vi "Begin.vi"(11 "Image Size":T1=enum."160x120") -> (0 "error out":errorcluster)   [LabVIEW 2011]
doc: "Called before other user functions, this VI is expected to open initial I/O refnums, load in file data, and do all program initialization. Notice that the <B>error out</B> terminal is simply used for data flow. Wiring it to other structures or subVIs ensures that this VI runs first."
uses:
  <vilib>/Rock Robotics/WPI/Camera/WPI_CameraImageSize.ctl
  <vilib>/Rock Robotics/SystemInterfaces/DIO/FPGA_DIOPWMChannel.ctl
  <vilib>/Rock Robotics/WPI/Joystick/WPI_JoystickDeviceEnum.ctl
  <vilib>/Rock Robotics/WPI/Camera/WPI_CameraWhite Balance Values.ctl
  <vilib>/Rock Robotics/WPI/Camera/WPI_CameraExposure Values.ctl
  <vilib>/Rock Robotics/WPI/Camera/WPI_CameraFrameRate.ctl
  <vilib>/Rock Robotics/SystemInterfaces/Typedef/FPGA_TypedefDigitalModule.ctl
  <vilib>/Rock Robotics/SystemInterfaces/Typedef/FPGA_TypedefAnalogModule.ctl
  <vilib>/Rock Robotics/SystemInterfaces/AI/FPGA_AIChannel.ctl
  <vilib>/Rock Robotics/SystemInterfaces/DIO/FPGA_DIOChannel.ctl
  <vilib>/Rock Robotics/SystemInterfaces/Typedef/FPGA_TypedefAnalogModuleForGyro.ctl
  <vilib>/Rock Robotics/SystemInterfaces/AI/FPGA_AIGyroChannel.ctl
  Common/ADXL345 I2C Range.ctl
  <vilib>/Rock Robotics/SystemInterfaces/DIO/FPGA_DIORelayChannel.ctl
  <vilib>/Rock Robotics/WPI/RobotDrive/WPI_RobotDriveOpen4MotorWithJaguar.vi
  <vilib>/Rock Robotics/WPI/MotorControl/WPI_MotorControlOpen Jaguar.vi
  <vilib>/Rock Robotics/WPI/Counter/WPI_CounterDigitalInputToDigitalSource.vi
  <vilib>/Rock Robotics/WPI/Counter/WPI_CounterOpen UpDown Mode.vi
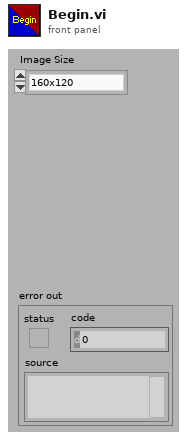
[diagram p1: front panel]
types:
  T1 = typedef "WPI_CameraImageSize.ctl" = enum16{"640x480", "320x240", "160x120"}
  T2 = typedef "FPGA_DIORelayChannel.ctl" = enum8{"Relay 1", "Relay 2", "Relay 3", "Relay 4", "Relay 5", "Relay 6", "Relay 7", "Relay 8", "Invalid"}
  T3 = typedef "FPGA_TypedefDigitalModule.ctl" = enum16{"Digital Module 1", "Digital Module 2"}
  T4 = typedef "FPGA_DIOChannel.ctl" = enum8{"DIO 1", "DIO 2", "DIO 3", "DIO 4", "DIO 5", "DIO 6", "DIO 7", "DIO 8", "DIO 9", "DIO 10", "DIO 11", "DIO 12", "DIO 13", "DIO 14", "Invalid"}
  T5 = typedef "FPGA_AIChannel.ctl" = enum8{"AI 1", "AI 2", "AI 3", "AI 4", "AI 5", "AI 6", "AI 7", "AI 8", "Invalid"}
  T6 = typedef "FPGA_TypedefAnalogModule.ctl" = enum16{"Analog Module 1", "Analog Module 2"}
  T7 = typedef "FPGA_DIOPWMChannel.ctl" = enum8{"PWM 1", "PWM 2", "PWM 3", "PWM 4", "PWM 5", "PWM 6", "PWM 7", "PWM 8", "PWM 9", "PWM 10", "Invalid"}
  T8 = typedef "ADXL345 I2C Range.ctl" = u8
  T9 = typedef "FPGA_AIGyroChannel.ctl" = enum8{"AI 1", "AI 2", "Invalid"}
  T10 = typedef "FPGA_TypedefAnalogModuleForGyro.ctl" = enum16{"Analog Module 1"}
  T11 = typedef "WPI_JoystickDeviceEnum.ctl" = enum16{"USB 1", "USB 2", "USB 3", "USB 4", "Kinect 1", "Kinect 2"}
  T12 = typedef "WPI_CameraFrameRate.ctl" = u32
  T13 = typedef "WPI_CameraExposure Values.ctl" = enum16{"Auto", "Flicker-free 50 Hz", "Flicker-free 60 Hz", "Hold current"}
  T14 = typedef "WPI_CameraWhite Balance Values.ctl" = enum16{"Auto", "Fixed indoor", "Fixed outdoor 1", "Fixed outdoor 2", "Fixed fluorescent 1", "Fixed fluorescent 2", "Hold current"}
  T15 = typedef "WPI_DigitalInputDevRef.ctl" = cluster{"DevStatus":errorcluster, "DIO Channel":T4, "Digital Module":T3}
  T16 = typedef "WPI_JoystickDevRef.ctl" = cluster{"Device":T11}
  T17 = typedef "WPI_AnalogChannelDevRef.ctl" = cluster{"DevStatus":errorcluster, "Analog Module":T6, "Analog Channel":T5}
  T18 = typedef "WPI_RobotDriveDevRef.ctl" = cluster{"DevStatus":errorcluster, "Motors[]":T19[], "Square Inputs":bool, "Max Output":dbl, "Isochronous":bool}
  T19 = typedef "WPI_MotorControlDeviceRef.ctl" = cluster{"DeviceStatus":errorcluster, "Type":enum16{"PWM", "CAN"}, "PWM":cluster{"Digital Module":T3, "PWM Channel":T7, "DeadBand":T20}, "CAN":cluster{"Device Number":u8, "Control Mode":T21, "Semaphore":T22, "Max Vout":dbl}, "Invert":bool, "TransformRef":T23, "InvTransformRef":T23}
  T20 = typedef "WPI_PWMDeadband.ctl" = cluster{"Name":string, "maxPositivePwm":i32, "minPositivePwm":i32, "centerPwm":i32, "maxNegativePwm":i32, "minNegativePwm":i32, "angularRange":u16}
  T21 = typedef "WPI_CANJaguar_ControlMode.ctl" = enum8{"Percent VBus", "Current", "Speed", "Position", "Voltage"}
  T22 = typedef "Semaphore RefNum" = refnum<k1>
  T23 = typedef "WPI_PWMTransform_ConPane.ctl" = refnum<vi>
  T24 = typedef "WPI_GyroDevRef.ctl" = cluster{"DevStatus":errorcluster, "Analog Module":T6, "Analog Channel":T5, "Offset":dbl, "Gain (VoltsPerDegree/Second)":dbl}
  T25 = typedef "WPI_I2CDevRef.ctl" = cluster{"DevStatus":errorcluster, "Digital Module":T3, "Device Address":u8}
  T26 = typedef "WPI_RelayDevRef.ctl" = cluster{"DevStatus":errorcluster, "Relay Channel":T2, "Digital Module":T3, "Relay Direction":T27}
  T27 = typedef "WPI_RelayDirection.ctl" = enum16{"Both directions", "Forward only", "Reverse only"}
  T28 = typedef "FPGA_CounterEncoderSourceConvertionLVSourceType.ctl" = cluster{"DevStatus":errorcluster, "AnalogTriggerMode?":bool, "DigitalMode":cluster{"Digital Module":T3, "DIO Channel":T29}, "AnalogTriggerMode":cluster{"AnalogTriggerIndex":T30, "OutputType":T31}}
  T29 = typedef "FPGA_DIODigitalSourceChannel.ctl" = enum8{"DIO 1", "DIO 2", "DIO 3", "DIO 4", "DIO 5", "DIO 6", "DIO 7", "DIO 8", "DIO 9", "DIO 10", "DIO 11", "DIO 12", "DIO 13", "DIO 14", "Disabled"}
  T30 = typedef "FPGA_AnalogTriggerIndex.ctl" = enum8{"Trig 0", "Trig 1", "Trig 2", "Trig 3", "Trig 4", "Trig 5", "Trig 6", "Trig 7", "Invalid"}
  T31 = typedef "FPGA_AnalogTriggerOutType.ctl" = enum16{"InWindow", "TriggerState", "Rising", "Falling"}
  T32 = typedef "WPI_EncoderDevRef.ctl" = cluster{"DevStatus":errorcluster, "EncoderIndex":T33, "CounterIndex":T34, "DistancePerCount":dbl, "Decoding Type":T35}
  T33 = typedef "FPGA_EncoderIdx.ctl" = enum8{"Enc 0", "Enc 1", "Enc 2", "Enc 3", "Invalid"}
  T34 = typedef "FPGA_CounterCtrSystemIndex.ctl" = enum8{"Ctr 0", "Ctr 1", "Ctr 2", "Ctr 3", "Ctr 4", "Ctr 5", "Ctr 6", "Ctr 7", "Invalid"}
  T35 = typedef "WPI_EncoderType.ctl" = enum16{"1x", "2x", "4x"}
  T36 = typedef "WPI_CounterDevRef.ctl" = cluster{"DevStatus":errorcluster, "CntIndex":T34}
  T37 = typedef "WPI_CameraDevRef.ctl" = cluster{"Camera Address":string, "CameraStatus":errorcluster, "Acquire Image Notifier":refnum<notifier>}
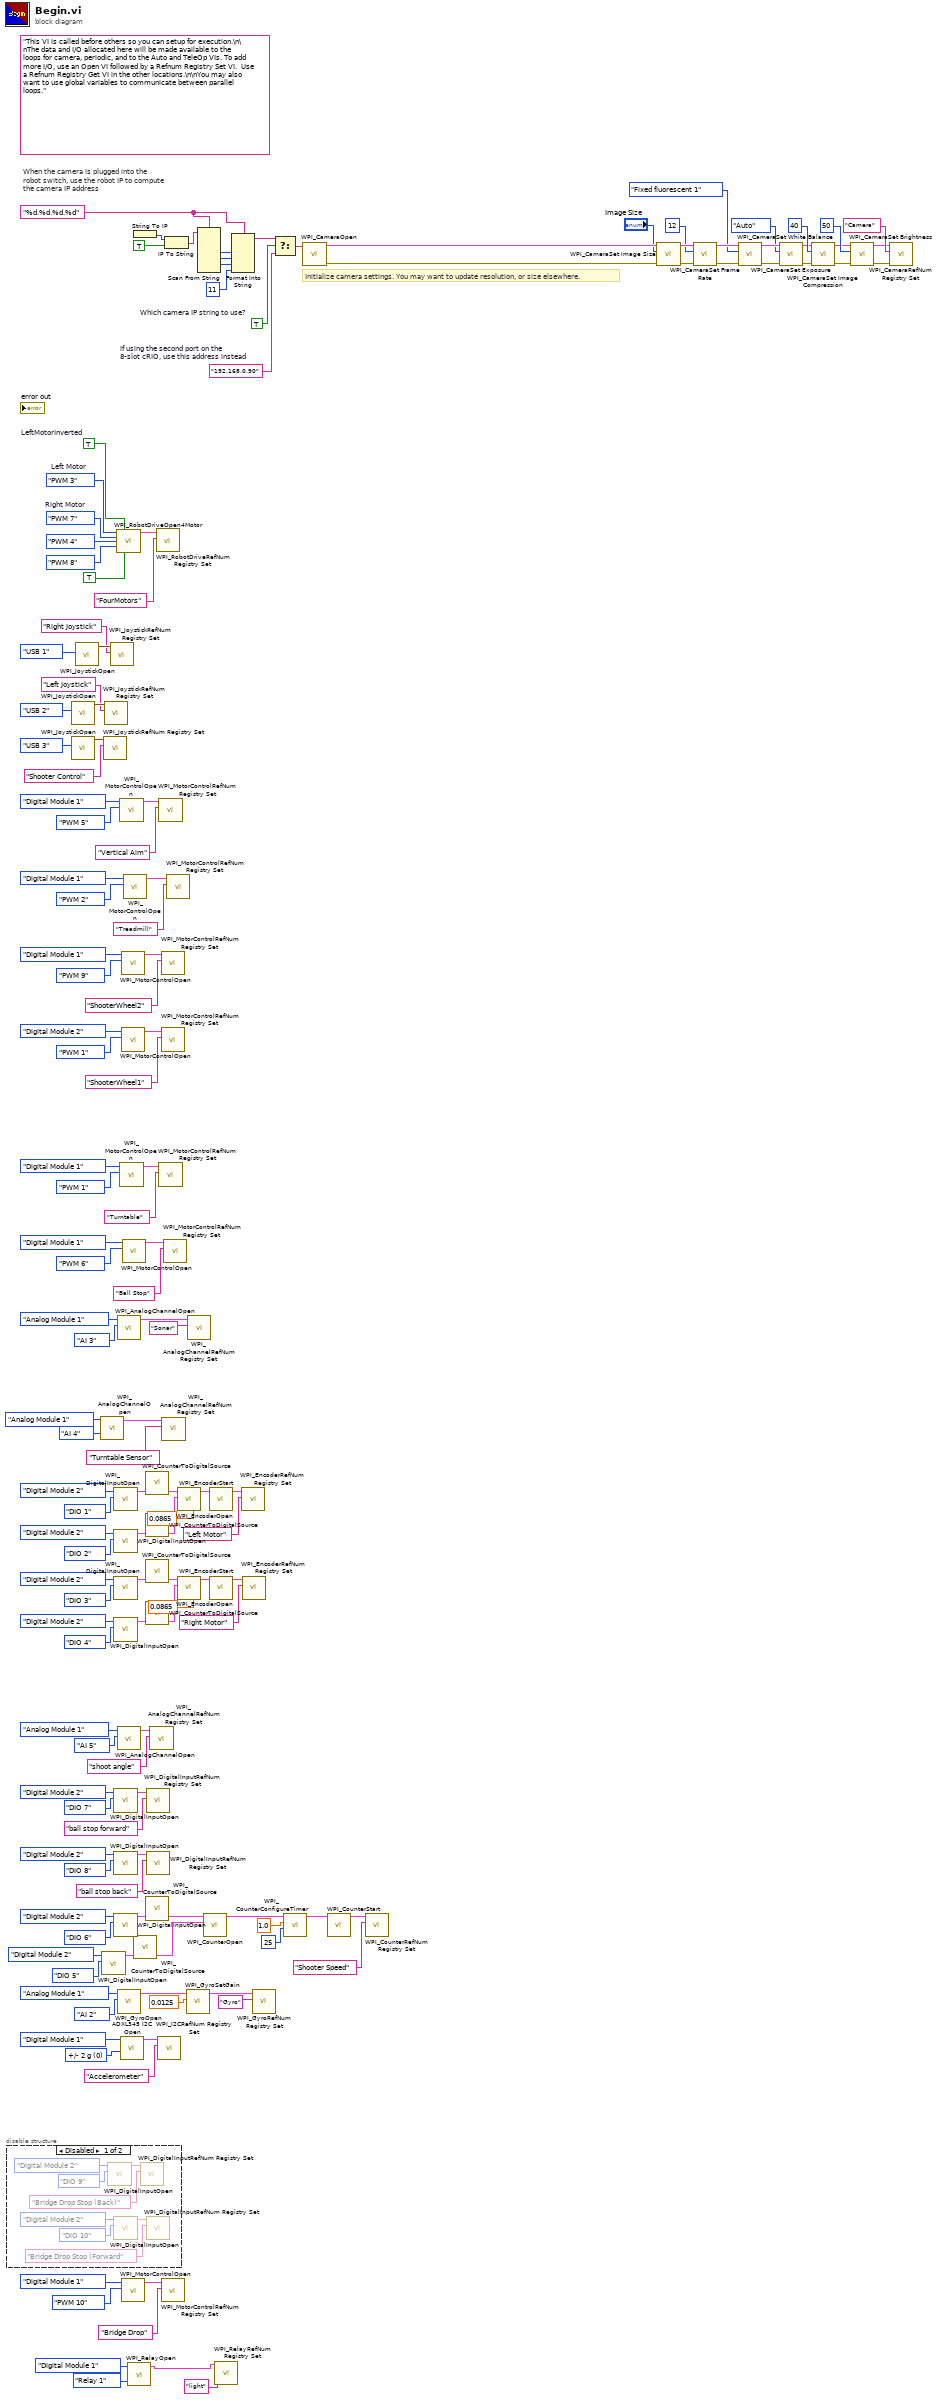
[diagram p0: block diagram]
diagram:
  w23 = T8 0 items=["+/- 2 g", "+/- 4 g", "+/- 8 g", "+/- 16 g"] ("Range")
  w110 = TRUE  # Which camera IP string to use?
  w114 = "%d.%d.%d.%d" ("format string")
  (unwired) "This VI is called before others so you can setup for execution.\n\nThe data and I/O allocated here will be made available to the loops for camera, periodic, and to the Auto and TeleOp VIs. To add more I/O, use an Open VI followed by a Refnum Registry Set VI.  Use a Refnum Registry Get VI in the other locations.\n\nYou may also want to use global variables to communicate between parallel loops."
  w126 = FPGA_DIOPWMChannel."PWM 7"  # Right Motor
  w127 = FPGA_DIOPWMChannel."PWM 3"  # Left Motor
  w111 = "192.168.0.90"  # If using the second port on the 8-slot cRIO, use this address instead
  w150 = TRUE  # LeftMotorInverted
  # "When the camera is plugged into the\nrobot switch, use the robot IP to compute\nthe camera IP address"
  # "Initialize camera settings. You may want to update resolution, or size elsewhere."
  n1 = disable-structure shown="Disabled" {
    frame Disabled {
      n2 = call <vilib>:"WPI_DigitalInputOpen.vi"("DIO Channel"=FPGA_DIOChannel."DIO 9", "Digital Module (Module 1)"=FPGA_TypedefDigitalModule."Digital Module 2") -> ("DigitalInputDevRef"=w151:T15)  [unwired: 8 in, 1 out]
      n3 = call <vilib>:"WPI_DigitalInputOpen.vi"("DIO Channel"=FPGA_DIOChannel."DIO 10", "Digital Module (Module 1)"=FPGA_TypedefDigitalModule."Digital Module 2") -> ("DigitalInputDevRef"=w158:T15)  [unwired: 8 in, 1 out]
      n4 = call <vilib>:"WPI_DigitalInputRefNum Registry Set.vi"("refnum name"="Bridge Drop Stop (Back)", "DigitalInputDevRef"=w151) -> ()  [unwired: 8 in, 2 out]
      n5 = call <vilib>:"WPI_DigitalInputRefNum Registry Set.vi"("refnum name"="Bridge Drop Stop (Forward", "DigitalInputDevRef"=w158) -> ()  [unwired: 8 in, 2 out]
    }
    frame Enabled {
    }
  }
  n6 = call <vilib>:"WPI_JoystickOpen.vi"("JoystickDevice"=WPI_JoystickDeviceEnum."USB 2") -> ("JoystickDevRef"=w109:T16)  [unwired: 10 in]
  n7 = call <vilib>:"WPI_JoystickOpen.vi"("JoystickDevice"=WPI_JoystickDeviceEnum."USB 3") -> ("JoystickDevRef"=w105:T16)  [unwired: 10 in]
  n8 = call <vilib>:"WPI_JoystickOpen.vi"("JoystickDevice"=WPI_JoystickDeviceEnum."USB 1") -> ("JoystickDevRef"=w146:T16)  [unwired: 10 out]
  n9 = call <vilib>:"WPI_AnalogChannelOpen.vi"("Analog Channel"=FPGA_AIChannel."AI 4", "Analog Module (Module 1)"=FPGA_TypedefAnalogModule."Analog Module 1") -> ("AIDeviceRef"=w14:T17)  [unwired: 8 in, 1 out]
  n10 = call <vilib>:"WPI_DigitalInputOpen.vi"("DIO Channel"=FPGA_DIOChannel."DIO 5", "Digital Module (Module 1)"=FPGA_TypedefDigitalModule."Digital Module 2") -> ("DigitalInputDevRef"=w10:T15)  [unwired: 8 in, 1 out]
  n11 = call <vilib>:"WPI_JoystickRefNum Registry Set.vi"("refnum name"="Shooter Control", "JoystickDevRef"=w105) -> ()  [unwired: 8 in, 2 out]
  n12 = call <vilib>:"WPI_JoystickRefNum Registry Set.vi"("refnum name"="Left Joystick", "JoystickDevRef"=w109) -> ()  [unwired: 8 in, 2 out]
  n13 = call <vilib>:"WPI_JoystickRefNum Registry Set.vi"("refnum name"="Right Joystick", "JoystickDevRef"=w146) -> ()  [unwired: 1 in, 9 out]
  n14 = call <vilib>:"WPI_DigitalInputOpen.vi"("DIO Channel"=FPGA_DIOChannel."DIO 1", "Digital Module (Module 1)"=FPGA_TypedefDigitalModule."Digital Module 2") -> ("DigitalInputDevRef"=w67:T15)  [unwired: 8 in, 1 out]
  n15 = call <vilib>:"WPI_DigitalInputOpen.vi"("DIO Channel"=FPGA_DIOChannel."DIO 2", "Digital Module (Module 1)"=FPGA_TypedefDigitalModule."Digital Module 2") -> ("DigitalInputDevRef"=w68:T15)  [unwired: 8 in, 1 out]
  n16 = call <vilib>:"WPI_DigitalInputOpen.vi"("DIO Channel"=FPGA_DIOChannel."DIO 3", "Digital Module (Module 1)"=FPGA_TypedefDigitalModule."Digital Module 2") -> ("DigitalInputDevRef"=w69:T15)  [unwired: 8 in, 1 out]
  n17 = call <vilib>:"WPI_DigitalInputOpen.vi"("DIO Channel"=FPGA_DIOChannel."DIO 4", "Digital Module (Module 1)"=FPGA_TypedefDigitalModule."Digital Module 2") -> ("DigitalInputDevRef"=w70:T15)  [unwired: 8 in, 1 out]
  n18 = call <vilib>:"WPI_DigitalInputOpen.vi"("DIO Channel"=FPGA_DIOChannel."DIO 7", "Digital Module (Module 1)"=FPGA_TypedefDigitalModule."Digital Module 2") -> ("DigitalInputDevRef"=w49:T15)  [unwired: 8 in, 1 out]
  n19 = call <vilib>:"WPI_DigitalInputOpen.vi"("DIO Channel"=FPGA_DIOChannel."DIO 8", "Digital Module (Module 1)"=FPGA_TypedefDigitalModule."Digital Module 2") -> ("DigitalInputDevRef"=w50:T15)  [unwired: 8 in, 1 out]
  n20 = call <vilib>:"WPI_DigitalInputOpen.vi"("DIO Channel"=FPGA_DIOChannel."DIO 6", "Digital Module (Module 1)"=FPGA_TypedefDigitalModule."Digital Module 2") -> ("DigitalInputDevRef"=w42:T15)  [unwired: 8 in, 1 out]
  n21 = call-poly <vilib>:"WPI_RobotDriveOpen4Motor.vi"("Rear Left Motor"=w127, "Rear Left Motor Inverted"=w150, "Rear Right Motor"=w126, "Front Left Motor"=FPGA_DIOPWMChannel."PWM 4", "Front Right Motor"=FPGA_DIOPWMChannel."PWM 8", "Front Left Motor Inverted"=TRUE) -> ("RobotDriveDevRef"=w148:T18)  [unwired: 8 in, 1 out]
  n22 = call <vilib>:"WPI_AnalogChannelOpen.vi"("Analog Channel"=FPGA_AIChannel."AI 3", "Analog Module (Module 1)"=FPGA_TypedefAnalogModule."Analog Module 1") -> ("AIDeviceRef"=w80:T17)  [unwired: 8 in, 1 out]
  n23 = call <vilib>:"WPI_AnalogChannelOpen.vi"("Analog Channel"=FPGA_AIChannel."AI 5", "Analog Module (Module 1)"=FPGA_TypedefAnalogModule."Analog Module 1") -> ("AIDeviceRef"=w52:T17)  [unwired: 8 in, 1 out]
  n24 = call <vilib>:"WPI_GyroOpen.vi"("Analog Channel"=FPGA_AIGyroChannel."AI 2", "Analog Module (Module 1)"=FPGA_TypedefAnalogModuleForGyro."Analog Module 1") -> ("GyroDevRef"=w32:T24)  [unwired: 4 in, 5 out]
  n25 = call-poly <vilib>:"WPI_MotorControlOpen.vi"("PWM Channel"=FPGA_DIOPWMChannel."PWM 5", "Digital Module (Module 1)"=FPGA_TypedefDigitalModule."Digital Module 1") -> ("MotorControlDeviceRef"=w100:T19)  [unwired: 8 in, 1 out]
  n26 = call-poly <vilib>:"WPI_MotorControlOpen.vi"("PWM Channel"=FPGA_DIOPWMChannel."PWM 1", "Digital Module (Module 1)"=FPGA_TypedefDigitalModule."Digital Module 1") -> ("MotorControlDeviceRef"=w82:T19)  [unwired: 8 in, 1 out]
  n27 = call "ADXL345 I2C Open.vi"("Range"=w23, "DIO Module (Slot 4)"=FPGA_TypedefDigitalModule."Digital Module 1") -> ("I2CDevRef"=w26:T25)  [unwired: 2 in, 7 out]
  n28 = call-poly <vilib>:"WPI_MotorControlOpen.vi"("PWM Channel"=FPGA_DIOPWMChannel."PWM 9", "Digital Module (Module 1)"=FPGA_TypedefDigitalModule."Digital Module 1") -> ("MotorControlDeviceRef"=w92:T19)  [unwired: 8 in, 1 out]
  n29 = call-poly <vilib>:"WPI_MotorControlOpen.vi"("PWM Channel"=FPGA_DIOPWMChannel."PWM 1", "Digital Module (Module 1)"=FPGA_TypedefDigitalModule."Digital Module 2") -> ("MotorControlDeviceRef"=w91:T19)  [unwired: 8 in, 1 out]
  n30 = call-poly <vilib>:"WPI_MotorControlOpen.vi"("PWM Channel"=FPGA_DIOPWMChannel."PWM 10", "Digital Module (Module 1)"=FPGA_TypedefDigitalModule."Digital Module 1") -> ("MotorControlDeviceRef"=w18:T19)  [unwired: 8 in, 1 out]
  n31 = call-poly <vilib>:"WPI_MotorControlOpen.vi"("PWM Channel"=FPGA_DIOPWMChannel."PWM 6", "Digital Module (Module 1)"=FPGA_TypedefDigitalModule."Digital Module 1") -> ("MotorControlDeviceRef"=w22:T19)  [unwired: 8 in, 1 out]
  n32 = call-poly <vilib>:"WPI_MotorControlOpen.vi"("PWM Channel"=FPGA_DIOPWMChannel."PWM 2", "Digital Module (Module 1)"=FPGA_TypedefDigitalModule."Digital Module 1") -> ("MotorControlDeviceRef"=w96:T19)  [unwired: 8 in, 1 out]
  n33 = call <vilib>:"WPI_RelayOpen.vi"("Relay Channel"=FPGA_DIORelayChannel."Relay 1", "Digital Module (Module 1)"=FPGA_TypedefDigitalModule."Digital Module 1") -> ("RelayDevRef"=w6:T26)  [unwired: 8 in, 1 out]
  n34 = String To IP() -> (0:w121:u32)  [unwired: 1 in]
  n35 = call-poly <vilib>:"WPI_CounterToDigitalSource.vi"("DigitalInputDevRef"=w10) -> ("Digital Source"=w7:T28)  [unwired: 6 in]
  n36 = call-poly <vilib>:"WPI_CounterToDigitalSource.vi"("DigitalInputDevRef"=w67) -> ("Digital Source"=w76:T28)  [unwired: 6 in]
  n37 = call-poly <vilib>:"WPI_CounterToDigitalSource.vi"("DigitalInputDevRef"=w68) -> ("Digital Source"=w75:T28)  [unwired: 6 in]
  n38 = call-poly <vilib>:"WPI_CounterToDigitalSource.vi"("DigitalInputDevRef"=w69) -> ("Digital Source"=w72:T28)  [unwired: 6 in]
  n39 = call-poly <vilib>:"WPI_CounterToDigitalSource.vi"("DigitalInputDevRef"=w70) -> ("Digital Source"=w71:T28)  [unwired: 6 in]
  n40 = call-poly <vilib>:"WPI_CounterToDigitalSource.vi"("DigitalInputDevRef"=w42) -> ("Digital Source"=w39:T28)  [unwired: 6 in]
  n41 = call <vilib>:"WPI_DigitalInputRefNum Registry Set.vi"("refnum name"="ball stop forward", "DigitalInputDevRef"=w49) -> ()  [unwired: 8 in, 2 out]
  n42 = call <vilib>:"WPI_DigitalInputRefNum Registry Set.vi"("refnum name"="ball stop back", "DigitalInputDevRef"=w50) -> ()  [unwired: 8 in, 2 out]
  n43 = call <vilib>:"WPI_AnalogChannelRefNum Registry Set.vi"("refnum name"="shoot angle", "AIDeviceRef"=w52) -> ()  [unwired: 8 in, 2 out]
  n44 = call <vilib>:"WPI_RobotDriveRefNum Registry Set.vi"("refnum name"="FourMotors", "RobotDriveDevRef"=w148) -> ()  [unwired: 1 in, 9 out]
  n45 = call <vilib>:"WPI_I2CRefNum Registry Set.vi"("refnum name"="Accelerometer", "I2CDevRef"=w26) -> ()  [unwired: 8 in, 2 out]
  n46 = call <vilib>:"WPI_MotorControlRefNum Registry Set.vi"("refnum name"="Vertical Aim", "MotorControlDevRef"=w100) -> ()  [unwired: 8 in, 2 out]
  n47 = call <vilib>:"WPI_MotorControlRefNum Registry Set.vi"("refnum name"="Turntable", "MotorControlDevRef"=w82) -> ()  [unwired: 8 in, 2 out]
  n48 = call <vilib>:"WPI_MotorControlRefNum Registry Set.vi"("refnum name"="ShooterWheel2", "MotorControlDevRef"=w92) -> ()  [unwired: 8 in, 2 out]
  n49 = call <vilib>:"WPI_MotorControlRefNum Registry Set.vi"("refnum name"="ShooterWheel1", "MotorControlDevRef"=w91) -> ()  [unwired: 8 in, 2 out]
  n50 = call <vilib>:"WPI_MotorControlRefNum Registry Set.vi"("refnum name"="Bridge Drop", "MotorControlDevRef"=w18) -> ()  [unwired: 8 in, 2 out]
  n51 = call <vilib>:"WPI_AnalogChannelRefNum Registry Set.vi"("refnum name"="Turntable Sensor", "AIDeviceRef"=w14) -> ()  [unwired: 8 in, 2 out]
  n52 = call <vilib>:"WPI_MotorControlRefNum Registry Set.vi"("refnum name"="Ball Stop", "MotorControlDevRef"=w22) -> ()  [unwired: 8 in, 2 out]
  n53 = IP To String(1:TRUE ("dot notation? (F)"), 2:w121) -> (0:w119:string)
  n54 = call <vilib>:"WPI_MotorControlRefNum Registry Set.vi"("refnum name"="Treadmill", "MotorControlDevRef"=w96) -> ()  [unwired: 8 in, 2 out]
  n55 = call <vilib>:"WPI_EncoderOpen.vi"("DistancePerCount"=0.0865, "BSource"=w75, "ASource"=w76) -> ("EncoderDevRef"=w73:T32)  [unwired: 7 in, 1 out]
  n56 = call <vilib>:"WPI_EncoderOpen.vi"("DistancePerCount"=0.0865, "BSource"=w71, "ASource"=w72) -> ("EncoderDevRef"=w74:T32)  [unwired: 7 in, 1 out]
  n57 = call <vilib>:"WPI_GyroSetGain.vi"("Gain (VoltsPerDegree/Second)"=0.0125, "GyroDevRef"=w32) -> ("GyroDevRef"=w28:T24)  [unwired: 1 in, 8 out]
  n58 = call <vilib>:"WPI_AnalogChannelRefNum Registry Set.vi"("refnum name"="Sonar", "AIDeviceRef"=w80) -> ()  [unwired: 8 in, 2 out]
  n59 = Scan From String(format string=w114, input string=w119) -> (output 1=w118:i32, output 2=w117:i32, output 3=w116:i32)  [unwired: 7 in, 3 out]
  n60 = call-poly <vilib>:"WPI_CounterOpen.vi"("Down Source"=w7, "Up Source"=w39) -> ("CounterDevRef"=w33:T36)  [unwired: 8 in, 1 out]
  n61 = call <vilib>:"WPI_EncoderStart.vi"("EncoderDevRef"=w73) -> ("EncoderDevRef"=w57:T32)  [unwired: 9 in, 1 out]
  n62 = call <vilib>:"WPI_EncoderStart.vi"("EncoderDevRef"=w74) -> ("EncoderDevRef"=w58:T32)  [unwired: 9 in, 1 out]
  n63 = call <vilib>:"WPI_RelayRefNum Registry Set.vi"("refnum name"="light", "RelayDevRef"=w6) -> ()  [unwired: 8 in, 2 out]
  n64 = Format Into String(format string=w114, w118, w117, w116, 11 ("Compression")) -> (resulting string=w112:string)  [unwired: 2 in, 1 out]
  n65 = call <vilib>:"WPI_EncoderRefNum Registry Set.vi"("refnum name"="Left Motor", "EncoderDevRef"=w57) -> ()  [unwired: 8 in, 2 out]
  n66 = call <vilib>:"WPI_EncoderRefNum Registry Set.vi"("refnum name"="Right Motor", "EncoderDevRef"=w58) -> ()  [unwired: 8 in, 2 out]
  n67 = call <vilib>:"WPI_GyroRefNum Registry Set.vi"("refnum name"="Gyro", "GyroDevRef"=w28) -> ()  [unwired: 8 in, 2 out]
  n68 = Select(t=w112, s=w110, f=w111) -> (s? t:f=w113:string)
  n69 = call <vilib>:"WPI_CounterConfigureTimer.vi"("Number Samples to Average"=u8 25, "MaxPeriod (sec)"=1.0, "CounterDevRef in"=w33) -> ("CounterDevRef out"=w37:T36)  [unwired: 7 in, 1 out]
  n70 = call <vilib>:"WPI_CameraOpen.vi"("Camera Address"=w113) -> ("error out"=w136:errorcluster, "CameraDevRef"=w137:T37)  [unwired: 1 in, 8 out]
  n71 = call <vilib>:"WPI_CounterStart.vi"("CounterDevRef in"=w37) -> ("CounterDevRef out"=w36:T36)  [unwired: 9 in, 1 out]
  n72 = call <vilib>:"WPI_CounterRefNum Registry Set.vi"("refnum name"="Shooter Speed", "CounterDevRef"=w36) -> ()  [unwired: 8 in, 2 out]
  n73 = call <vilib>:"WPI_CameraSet Image Size.vi"("error in (no error)"=w136, "Image Size"="Image Size", "CameraDevRef"=w137) -> ("error out"=w135:errorcluster, "CameraDevRef Out"=w138:T37)  [unwired: 7 out]
  n74 = call <vilib>:"WPI_CameraSet Frame Rate.vi"("error in (no error)"=w135, "Frame Rate (fps)"=T12 12, "CameraDevRef"=w138) -> ("error out"=w134:errorcluster, "CameraDevRef Out"=w140:T37)  [unwired: 7 out]
  n75 = call <vilib>:"WPI_CameraSet White Balance.vi"("error in (no error)"=w134, "White Balance"=WPI_CameraWhite_Balance_Values."Fixed fluorescent 1", "CameraDevRef"=w140) -> ("error out"=w133:errorcluster, "CameraDevRef Out"=w139:T37)  [unwired: 7 out]
  n76 = call <vilib>:"WPI_CameraSet Exposure.vi"("error in (no error)"=w133, "Exposure"=WPI_CameraExposure_Values."Auto", "CameraDevRef"=w139) -> ("error out"=w132:errorcluster, "CameraDevRef Out"=w142:T37)  [unwired: 7 out]
  n77 = call <vilib>:"WPI_CameraSet Image Compression.vi"("error in (no error)"=w132, "Compression"=40, "CameraDevRef"=w142) -> ("error out"=w131:errorcluster, "CameraDevRef Out"=w141:T37)  [unwired: 7 out]
  n78 = call <vilib>:"WPI_CameraSet Brightness.vi"("error in (no error)"=w131, "Brightness"=50, "CameraDevRef"=w141) -> ("error out"=w129:errorcluster, "CameraDevRef Out"=w130:T37)  [unwired: 7 out]
  n79 = call <vilib>:"WPI_CameraRefNum Registry Set.vi"("error in (no error)"=w129, "refnum name"="Camera", "CameraDevRef"=w130) -> ()  [unwired: 9 out]
